vi "Input Dialog Box.vi"(0 "Current Input":i32, 2 "Edit?":bool, 7 "Input Array_Edit":u8[](array[numeric]), 11 "Input Array_All":u8[][](array[numeric])) -> (4 "Numeric Array":u8[](array[numeric]), 6 "String Array":string[](array[string]), 8 "Cancel Out":bool)   [LabVIEW 2010]
panel:
  in  "OK":bool
  in  "Cancel":bool
  in  "Type":T1(ring)
  in  "Module":T2(ring)
  in  "Input Channel":u8(ring)
  # "Main Configuration"
  # "Module Configuration"
  # "Input Parameters"
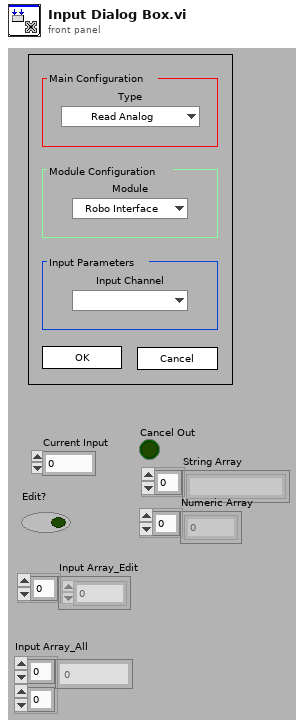
[diagram p1: front panel]
types:
  T1 = enum16{"Read Analog", "Read Digital", "Read Digital Distance"}
  T2 = enum8{"Robo Interface", "Extension 1", "Extension 2", "Extension 3"}
  T3 = typedef "LVStringsAndValuesArrayTypeDef.ctl" = cluster{"String":string, "Value":u8}[]
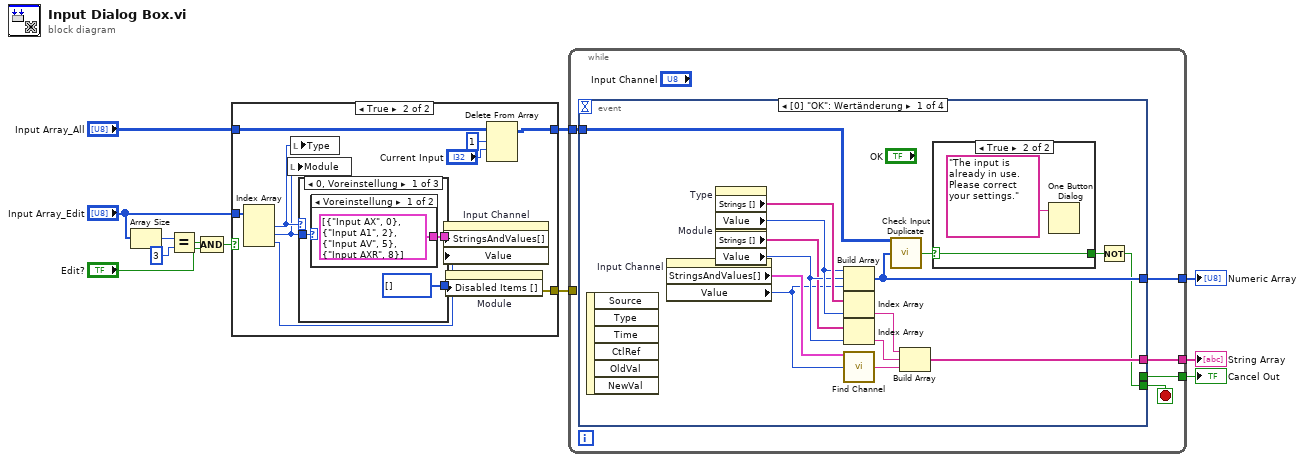
[diagram p0: block diagram]
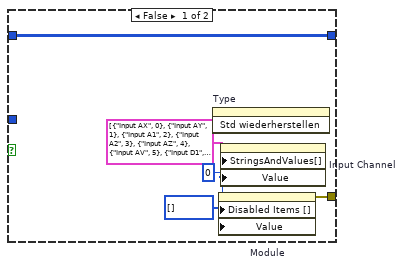
[diagram p2: hidden frame]
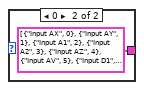
[diagram p3: hidden frame]
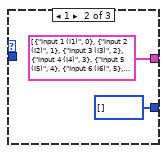
[diagram p4: hidden frame]
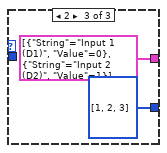
[diagram p5: hidden frame]
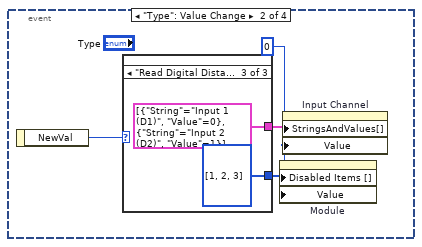
[diagram p7: hidden frame]
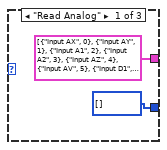
[diagram p8: hidden frame]
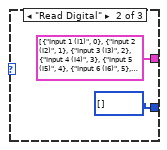
[diagram p9: hidden frame]
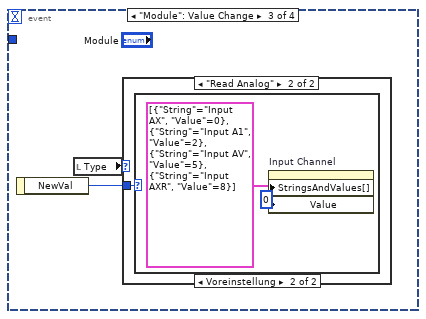
[diagram p10: hidden frame]
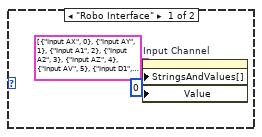
[diagram p12: hidden frame]
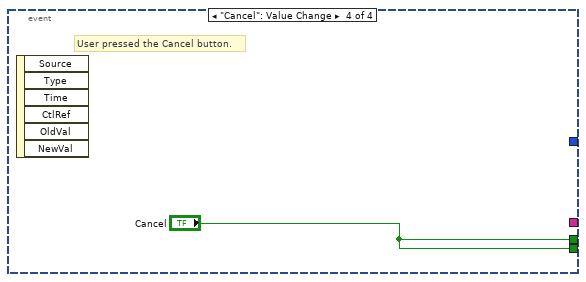
[diagram p13: hidden frame]
diagram:
  n1 = Array Size(array="Input Array_Edit") -> (size(s)=w7:i32)
  n2 = Equal?(x=w7, y=3) -> (x = y?=w10:bool)
  n3 = Compound Arithmetic op=AND(w10, "Edit?") -> (w8:bool)
  n4 = case shown="True" w8 {
    tunnel: "Input Array_Edit" -> [_ w28]
    tunnel: [w15 w24] -> w3
    tunnel: "Input Array_All" -> [w13 w22]
    tunnel: [w13 w21] -> w1
    frame False {
      w14 = u8 0
      n5 = invoke on="Type" class="Enum (strict)" method="Std wiederherstellen"() -> ()  [unwired: 3 in, 3 out]
      n6 = property on="Module" class="Enum (strikt)"("Disabled Items []"=i32[] [], "Value"=w14) -> (error out=w15:errorcluster)  [unwired: 2 in, 1 out]
      n7 = property on="Input Channel" class="Ring (strikt)"("StringsAndValues[]"=cluster{"String":string, "Value":u8}[] [{"String"="Input AX", "Value"=0}, {"String"="Input AY", "Value"=1}, {"String"="Input A1", "Value"=2}, {"String"="Input A2", "Value"=3}, {"String"="Input AZ", "Value"=4}, {"String"="Input AV", "Value"=5}, {"String"="Input D1", "Value"=6}, {"String"="Input D2", "Value"=7}, {"String"="Input AXR", "Value"=8}, {"String"="Input AYR", "Value"=9}] ("Strings And Values []"), "Value"=w14) -> ()  [unwired: 2 in, 2 out]
    }
    frame True {
      n8 = Index Array(array=w28) -> (element #1=w27:u8, element #2=w18:u8, element #3=w23:u8)  [unwired: 3 in]
      n9 = local write "Module"(w18) -> ()
      n10 = local write "Type"(w27) -> ()
      n11 = case shown="0, Voreinstellung" w27 {
        tunnel: [w30 cluster{"String":string, "Value":u8}[] [{"String"="Input 1 (I1)", "Value"=0}, {"String"="Input 2 (I2)", "Value"=1}, {"String"="Input 3 (I3)", "Value"=2}, {"String"="Input 4 (I4)", "Value"=3}, {"String"="Input 5 (I5)", "Value"=4}, {"String"="Input 6 (I6)", "Value"=5}, {"String"="Input 7 (I7)", "Value"=6}, {"String"="Input 8 (I8)", "Value"=7}] ("Strings And Values []") cluster{"String":string, "Value":u8}[] [{"String"="Input 1 (D1)", "Value"=0}, {"String"="Input 2 (D2)", "Value"=1}] ("Strings And Values []")] -> w26
        tunnel: [i32[] [] ("Disabled Items []") i32[] [] ("Disabled Items []") i32[] [1, 2, 3] ("Disabled Items []")] -> w25
        tunnel: w18 -> [w29 _ _]
        frame 0, Default {
          n12 = case shown="Voreinstellung" w29 {
            tunnel: [cluster{"String":string, "Value":u8}[] [{"String"="Input AX", "Value"=0}, {"String"="Input A1", "Value"=2}, {"String"="Input AV", "Value"=5}, {"String"="Input AXR", "Value"=8}] ("Strings And Values []") cluster{"String":string, "Value":u8}[] [{"String"="Input AX", "Value"=0}, {"String"="Input AY", "Value"=1}, {"String"="Input A1", "Value"=2}, {"String"="Input A2", "Value"=3}, {"String"="Input AZ", "Value"=4}, {"String"="Input AV", "Value"=5}, {"String"="Input D1", "Value"=6}, {"String"="Input D2", "Value"=7}, {"String"="Input AXR", "Value"=8}, {"String"="Input AYR", "Value"=9}] ("Strings And Values []")] -> w30
            frame Default {
            }
            frame 0 {
            }
          }
        }
        frame 1 {
        }
        frame 2 {
        }
      }
      n13 = property on="Input Channel" class="Ring (strikt)"("StringsAndValues[]"=w26, "Value"=w23) -> ()  [unwired: 2 in, 2 out]
      n14 = property on="Module" class="Enum (strikt)"("Disabled Items []"=w25) -> (error out=w24:errorcluster)  [unwired: 2 in, 1 out]
      n15 = Delete From Array(array=w22, length=1, index (row)="Current Input") -> (array with subset deleted=w21:u8[][])  [unwired: 1 in, 1 out]
    }
  }
  n16 = while {
    tunnel: [w41] -> w12
    tunnel: w3 -> [_]
    tunnel: [w40] -> w5
    tunnel: [w39] -> w4
    tunnel: w1 -> [w38]
    stop <- w42 stop-if-true
    n17 = event shown="[0] \"OK\": Wertänderung" {
      selector: _ -> [_ _ _ _]
      dyn-events: _ -> [_ _ _ _]
      timeout: _ -> [_ _ _ _]
      tunnel: [w51 _ _ "Cancel"] -> w42
      tunnel: [_ _ _ "Cancel"] -> w41
      tunnel: [w54 _ _ _] -> w40
      tunnel: [w55 _ _ _] -> w39
      tunnel: w38 -> [w46 _ _ _]
      event "OK": Value Change {
        n18 = event-data() -> ()  [unwired: 1 in, 6 out]
        n19 = property on="Input Channel" class="Ring (strikt)"() -> ("StringsAndValues[]"=w45:T3, "Value"=w44:u8)  [unwired: 2 in, 2 out]
        n20 = property on="Type" class="Enum (strikt)"() -> ("Strings []"=w50:string[], "Value"=w49:T1)  [unwired: 2 in, 2 out]
        n21 = property on="Module" class="Enum (strikt)"() -> ("Strings []"=w47:string[], "Value"=w48:T2)  [unwired: 2 in, 2 out]
        n22 = Build Array(w49, w48, w44) -> (w54:u16[])
        n23 = Index Array(array=w50, index=w49) -> (element=w56:string)
        n24 = Index Array(array=w47, index=w48) -> (element=w57:string)
        n25 = call "Find Channel.vi"("Strings And Values []"=w45, "Value"=w44) -> ("Channel"=w43:string)  [unwired: 13 in]
        n26 = call "Check Input Duplicate.vi"("Input Array"=w46, "New Point"=w54) -> ("Duplicate?"=w53:bool)  [unwired: 13 in]
        n27 = Build Array(w56, w57, w43) -> (w55:string[])
        n28 = case shown="True" w53 {
          selector: w53 -> [w58 w59]
          tunnel: [w58 w59] -> w52
          frame False {
          }
          frame True {
            n29 = One Button Dialog(message="The input is already in use.  Please correct your settings.") -> ()  [unwired: 1 in, 1 out]
          }
        }
        n30 = Not(x=w52) -> (.not. x?=w51:bool)
      }
      event "Type": Value Change {
        w64 = u8 0
        n31 = event-data() -> ("NewVal"=w61:T1)  [unwired: 1 in]
        n32 = case shown="\"Read Digital Distance\"" w61 {
          tunnel: [cluster{"String":string, "Value":u8}[] [{"String"="Input AX", "Value"=0}, {"String"="Input AY", "Value"=1}, {"String"="Input A1", "Value"=2}, {"String"="Input A2", "Value"=3}, {"String"="Input AZ", "Value"=4}, {"String"="Input AV", "Value"=5}, {"String"="Input D1", "Value"=6}, {"String"="Input D2", "Value"=7}, {"String"="Input AXR", "Value"=8}, {"String"="Input AYR", "Value"=9}] ("Strings And Values []") cluster{"String":string, "Value":u8}[] [{"String"="Input 1 (I1)", "Value"=0}, {"String"="Input 2 (I2)", "Value"=1}, {"String"="Input 3 (I3)", "Value"=2}, {"String"="Input 4 (I4)", "Value"=3}, {"String"="Input 5 (I5)", "Value"=4}, {"String"="Input 6 (I6)", "Value"=5}, {"String"="Input 7 (I7)", "Value"=6}, {"String"="Input 8 (I8)", "Value"=7}] ("Strings And Values []") cluster{"String":string, "Value":u8}[] [{"String"="Input 1 (D1)", "Value"=0}, {"String"="Input 2 (D2)", "Value"=1}] ("Strings And Values []")] -> w63
          tunnel: [i32[] [] ("Disabled Items []") i32[] [] ("Disabled Items []") i32[] [1, 2, 3] ("Disabled Items []")] -> w62
          frame "Read Analog" {
          }
          frame "Read Digital" {
          }
          frame "Read Digital Distance" {
          }
        }
        n33 = property on="Module" class="Enum (strikt)"("Disabled Items []"=w62, "Value"=w64) -> ()  [unwired: 2 in, 2 out]
        n34 = property on="Input Channel" class="Ring (strikt)"("StringsAndValues[]"=w63, "Value"=w64) -> ()  [unwired: 2 in, 2 out]
      }
      event "Module": Value Change {
        n35 = event-data() -> ("NewVal"=w72:T2)  [unwired: 1 in]
        n36 = local read "Type"() -> (w71:T1)
        n37 = case shown="\"Read Analog\"" w71 {
          tunnel: w72 -> [_ w73]
          frame Default {
          }
          frame "Read Analog" {
            n38 = case shown="Voreinstellung" w73 {
              frame "Robo Interface" {
                n39 = property on="Input Channel" class="Ring (strikt)"("StringsAndValues[]"=cluster{"String":string, "Value":u8}[] [{"String"="Input AX", "Value"=0}, {"String"="Input AY", "Value"=1}, {"String"="Input A1", "Value"=2}, {"String"="Input A2", "Value"=3}, {"String"="Input AZ", "Value"=4}, {"String"="Input AV", "Value"=5}, {"String"="Input D1", "Value"=6}, {"String"="Input D2", "Value"=7}, {"String"="Input AXR", "Value"=8}, {"String"="Input AYR", "Value"=9}] ("Strings And Values []"), "Value"=u8 0) -> ()  [unwired: 2 in, 2 out]
              }
              frame Default {
                n40 = property on="Input Channel" class="Ring (strikt)"("StringsAndValues[]"=cluster{"String":string, "Value":u8}[] [{"String"="Input AX", "Value"=0}, {"String"="Input A1", "Value"=2}, {"String"="Input AV", "Value"=5}, {"String"="Input AXR", "Value"=8}] ("Strings And Values []"), "Value"=u8 0) -> ()  [unwired: 2 in, 2 out]
              }
            }
          }
        }
      }
      event "Cancel": Value Change {
        # "User pressed the Cancel button."
        n41 = event-data() -> ()  [unwired: 1 in, 6 out]
      }
    }
  }
  "Cancel Out" <- w12
  "String Array" <- w4
  "Numeric Array" <- w5
